vi "SetLibraryFullState.vi"(8 "error in (no error)":errorcluster, 9 "Full":bool, 10 "LibraryPK":i32, 11 "Connection in":refnum<class "Connection.lvclass">) -> (0 "error out":errorcluster, 3 "Connection out":refnum<class "Connection.lvclass">)   [LabVIEW 2018, in "ErrorDefinitionSQLite.lvclass"]
uses:
  ErrorDefinitionSQLite.lvclass
  <vilib>/drjdpowell/SQLite Library/SQL Connection/Connection.lvclass
  <vilib>/drjdpowell/SQLite Library/SQL Connection/Execute SQL.vi
  <vilib>/drjdpowell/SQLite Library/SQLite.lvlib
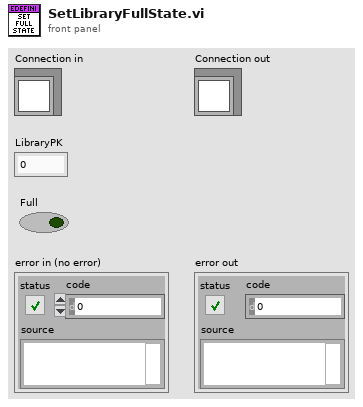
[diagram p1: front panel]
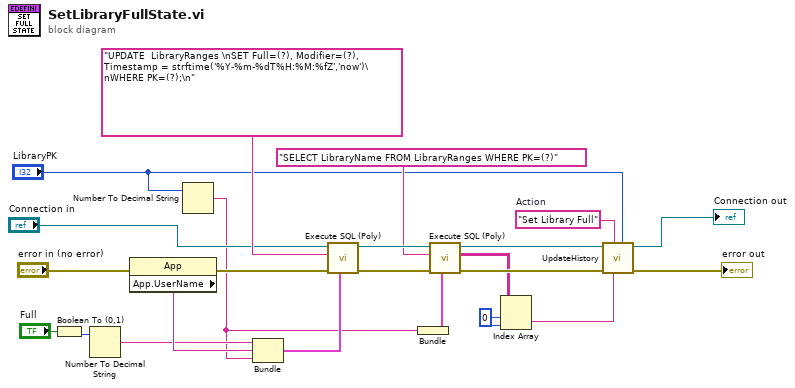
[diagram p0: block diagram]
diagram:
  w4 = 0 ("index (row)")
  w12 = "Set Library Full"  # Action
  n1 = Boolean To (0,1)(Boolean="Full") -> (0, 1=w16:i16)
  n2 = Number To Decimal String(number=w16) -> (decimal integer string=w15:string)  [unwired: 1 in]
  n3 = property class="App"(error in="error in (no error)") -> (error out=w23:errorcluster, "App.UserName"=w18:string)  [unwired: 1 in, 1 out]
  n4 = Number To Decimal String(number="LibraryPK") -> (decimal integer string=w1:string)  [unwired: 1 in]
  n5 = Bundle(w15, "App.UserName"=w18, w1) -> (w21:cluster{string, "App.UserName":string, string})  [unwired: 1 in]
  n6 = call-poly <vilib>:"Execute SQL (Poly).vi"("Parameter(s)"=w21, "error in (no error)"=w23, "SQL"="UPDATE  LibraryRanges \nSET Full=(?), Modifier=(?), Timestamp = strftime('%Y-%m-%dT%H:%M:%fZ','now')\nWHERE PK=(?);\n", "SQLite Connection in"="Connection in") -> ("error out"=w10:errorcluster, "SQLite Connection"=w11:refnum<class "Connection.lvclass">)  [unwired: 4 in, 2 out]
  n7 = Bundle(w1) -> (w7:cluster{string})  [unwired: 1 in]
  n8 = call-poly <vilib>:"Execute SQL (Poly).vi"("Parameter(s)"=w7, "error in (no error)"=w10, "SQL"="SELECT LibraryName FROM LibraryRanges WHERE PK=(?)", "SQLite Connection in"=w11) -> ("error out"=w6:errorcluster, "Result Set"=w5:string[][], "SQLite Connection"=w2:refnum<class "Connection.lvclass">)  [unwired: 4 in, 1 out]
  n9 = Index Array(array=w5, index (row)=w4, index (col)=w4) -> (element=w3:string)
  n10 = call "UpdateHistory.vi"("LibraryPK"="LibraryPK", "Library"=w3, "Action"=w12, "error in (no error)"=w6, "Connection in"=w2) -> ("error out"=→"error out":errorcluster, "Connection out"=→"Connection out":refnum<class "Connection.lvclass">)  [unwired: 5 in]
